vi "Update PID Parameters in System Definition.vi"(7 "Name":string, 8 "error in (no error)":errorcluster, 9 "Parameters":T1, 10 "NIVS SysDefRoot Ref":refnum<k24>, 11 "NIVS SysDef Ref":refnum<k24>) -> (0 "error out":errorcluster)   [LabVIEW 2019, in "Control Workspace Tool.lvlib"]
uses:
  Control Workspace Tool.lvlib
  NationalInstruments.VeriStand.SystemStorage
  Addon/Addon Shared/Types/Update Parameters Message.ctl
  NationalInstruments.VeriStand.SystemDefinitionAPI
  Addon/Addon Shared/SubVIs/Constants.vi
  Addon/Addon Shared/Control Addon Shared.lvlib
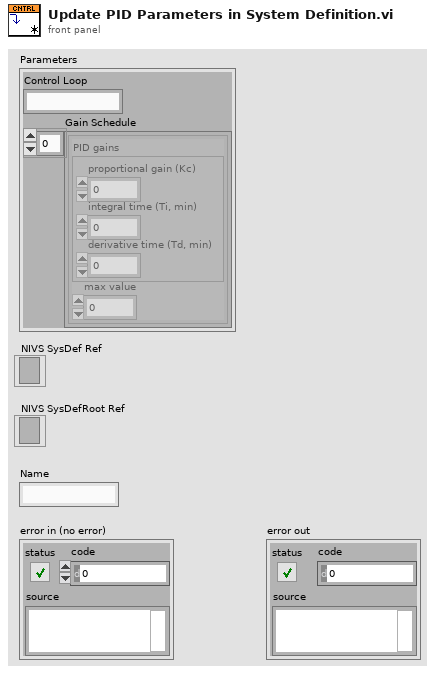
[diagram p1: front panel]
types:
  T1 = typedef "Control Addon Shared.lvlib/Update Parameters Message.ctl" = cluster{"Control Loop":string, "Gain Schedule":cluster{"PID gains":cluster{"proportional gain (Kc)":dbl, "integral time (Ti, min)":dbl, "derivative time (Td, min)":dbl}, "max value":dbl}[]}
  T2 = cluster{"PID gains":cluster{"proportional gain (Kc)":dbl, "integral time (Ti, min)":dbl, "derivative time (Td, min)":dbl}, "max value":dbl}[]
  T3 = cluster{"proportional gain (Kc)":dbl, "integral time (Ti, min)":dbl, "derivative time (Td, min)":dbl}
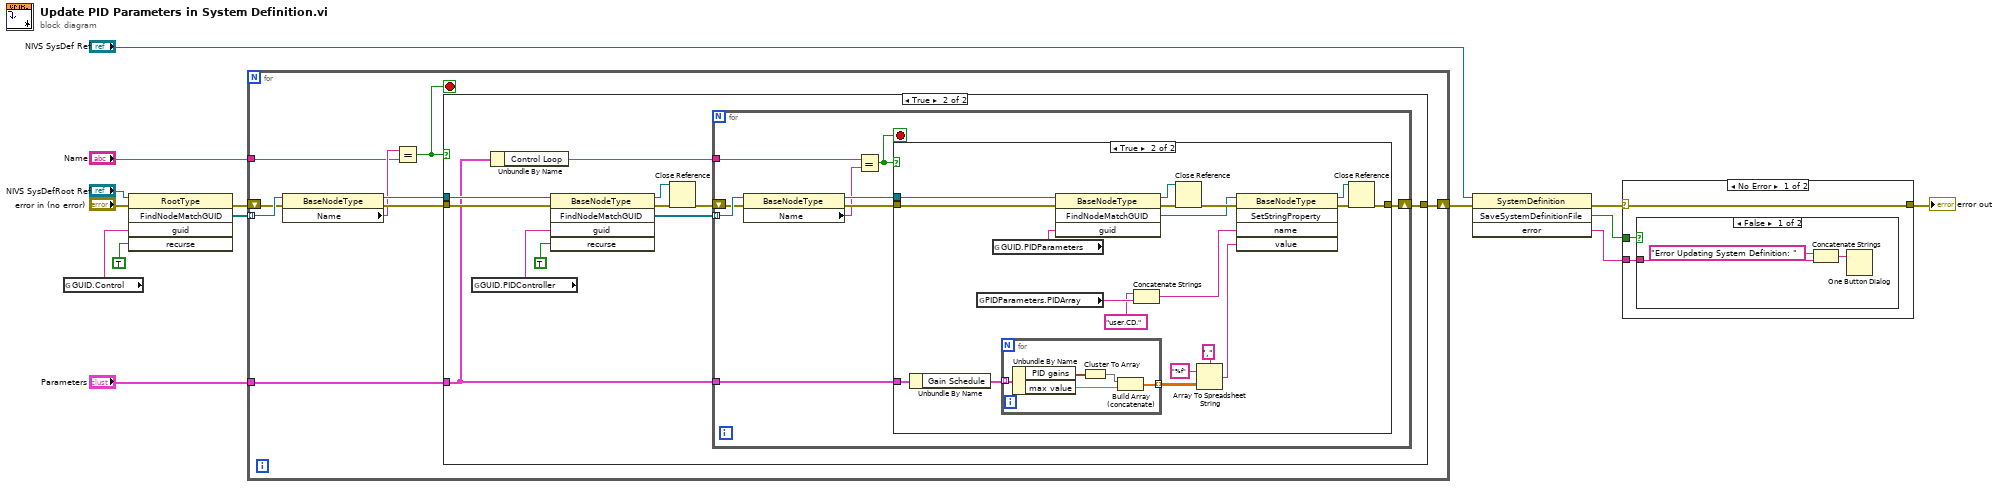
[diagram p0: block diagram]
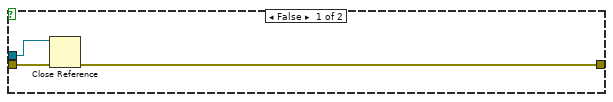
[diagram p5: hidden frame]
diagram:
  n1 = global read "Constants.vi" "GUID.Control"() -> (w10:string)
  n2 = invoke class="RootType" method="FindNodeMatchGUID"(reference="NIVS SysDefRoot Ref", error in="error in (no error)", "guid"=w10, "recurse"=TRUE) -> (error out=w14:errorcluster, "FindNodeMatchGUID"=w13:refnum<k24>[])  [unwired: 1 in, 3 out]
  n3 = for {
    tunnel: "Parameters" -> [w20]
    shift-right: [w23] -> w6
    shift-left: w14 -> [w21]
    tunnel: w13 -> [w22] mode=indexing
    tunnel: "Name" -> [w15]
    stop <- w19 stop-if-true
    n4 = property class="BaseNodeType"(reference=w22, error in=w21) -> (reference out=w17:refnum<k24>, error out=w18:errorcluster, "Name"=w16:string)
    n5 = Equal?(x=w16, y=w15) -> (x = y?=w19:bool)
    n6 = case shown="True" w19 {
      tunnel: [w24 w32] -> w23
      tunnel: w17 -> [_ w31]
      tunnel: w18 -> [w24 w30]
      tunnel: w20 -> [_ w26]
      frame False {
      }
      frame True {
        n7 = global read "Constants.vi" "GUID.PIDController"() -> (w35:string)
        n8 = Unbundle By Name(w26) -> ("Control Loop"=w25:string)
        n9 = invoke class="BaseNodeType" method="FindNodeMatchGUID"(reference=w31, error in=w30, "guid"=w35, "recurse"=TRUE) -> (reference out=w29:refnum<k24>, error out=w28:errorcluster, "FindNodeMatchGUID"=w33:refnum<k24>[])  [unwired: 1 in, 2 out]
        n10 = Close Reference(reference=w29, error in (no error)=w28) -> (error out=w27:errorcluster)
        n11 = for {
          tunnel: w33 -> [w43] mode=indexing
          shift-right: [w39] -> w32
          shift-left: w27 -> [w42]
          tunnel: w26 -> [w44]
          tunnel: w25 -> [w36]
          stop <- w38 stop-if-true
          n12 = property class="BaseNodeType"(reference=w43, error in=w42) -> (reference out=w41:refnum<k24>, error out=w40:errorcluster, "Name"=w37:string)
          n13 = Equal?(x=w36, y=w37) -> (x = y?=w38:bool)
          n14 = case shown="True" w38 {
            tunnel: w44 -> [_ w59]
            tunnel: w41 -> [w47 w57]
            tunnel: w40 -> [w46 w56]
            tunnel: [w45 w53] -> w39
            frame False {
              n15 = Close Reference(reference=w47, error in (no error)=w46) -> (error out=w45:errorcluster)
            }
            frame True {
              n16 = Unbundle By Name(w59) -> ("Gain Schedule"=w50:T2)
              n17 = global read "Constants.vi" "PIDParameters.PIDArray"() -> (w62:string)
              n18 = global read "Constants.vi" "GUID.PIDParameters"() -> (w66:string)
              n19 = for {
                tunnel: w50 -> [w71] mode=indexing
                tunnel: [w67] -> w49 mode=indexing
                n20 = Unbundle By Name(w71) -> ("PID gains"=w70:T3, "max value"=w68:dbl)
                n21 = Cluster To Array(cluster=w70) -> (array=w69:dbl[])
                n22 = Build Array (concatenate)(w69, w68) -> (w67:dbl[])
              }
              n23 = invoke class="BaseNodeType" method="FindNodeMatchGUID"(reference=w57, error in=w56, "guid"=w66) -> (reference out=w61:refnum<k24>, error out=w60:errorcluster, "FindNodeMatchGUID"=w51:refnum<k24>)  [unwired: 1 in, 1 out]
              n24 = Concatenate Strings("user.CD." ("string"), w62) -> (w48:string)
              n25 = Close Reference(reference=w61, error in (no error)=w60) -> (error out=w52:errorcluster)
              n26 = Array To Spreadsheet String(delimiter (Tab)=",", array=w49, 3:"%f" ("format string")) -> (spreadsheet string=w63:string)
              n27 = invoke class="BaseNodeType" method="SetStringProperty"(reference=w51, error in=w52, "name"=w48, "value"=w63) -> (reference out=w54:refnum<k24>, error out=w55:errorcluster)  [unwired: 1 in, 3 out]
              n28 = Close Reference(reference=w54, error in (no error)=w55) -> (error out=w53:errorcluster)
            }
          }
        }
      }
    }
  }
  n29 = invoke class="SystemDefinition" method="SaveSystemDefinitionFile"(reference="NIVS SysDef Ref", error in=w6) -> (error out=w2:errorcluster, "SaveSystemDefinitionFile"=w3:bool, "error"=w4:string)  [unwired: 2 in, 1 out]
  n30 = case shown="No Error" w2 {
    selector: w2 -> [w72 w78]
    tunnel: w4 -> [w74 _]
    tunnel: w3 -> [w73 _]
    tunnel: [w72 w78] -> w1
    frame No Error {
      n31 = case shown="False" w73 {
        tunnel: w74 -> [w77 _]
        frame False {
          n32 = Concatenate Strings("Error Updating System Definition: " ("string"), w77) -> (w76:string)
          n33 = One Button Dialog(message=w76) -> ()  [unwired: 1 in, 1 out]
        }
        frame True {
        }
      }
    }
    frame Error {
    }
  }
  "error out" <- w1
